vi "Stream User Timestamps to Disk.vi"(0 "fpga interface in":refnum<k20>, 5 "'stop' notifier":refnum<notifier>, 7 "base tdms file path":path, 9 "fetch size (elements)":u32=4096, 11 "error in (no error)":errorcluster) -> (4 "fpga interface out":refnum<k20>, 6 "file path out":path, 8 "gpio timestamp fifo overflow":bool, 15 "error out":errorcluster)   [LabVIEW 2023, in "GettingStarted_Common_148X_Host.lvlib"]
uses:
  GettingStarted_Common_148X_Host.lvlib
  Types/148x_Common_FPGA_Reference.ctl
  <vilib>/Utility/error.llb/Error Cluster From Error Code.vi
  <vilib>/rvi/errors/niLvFpgaAdjustHostInterfaceError.vi
  <vilib>/rvi/interface/nirviMethod/nirviMethod.xnode
  <vilib>/rvi/interface/nirviReadWriteControl/nirviReadWriteControl.xnode
  <vilib>/FPGAPlugInAG/Dynamic/niLvFpga_AcquireReadRegionFifo_Dynamic.vi
  <vilib>/rvi/errors/niLvFpgaMergeErrorWithErrorCode.vi
  NiFpgaLv.dll
  <vilib>/rvi/interface/Simulation/niFpgaSimulationCallBeginRW.vi
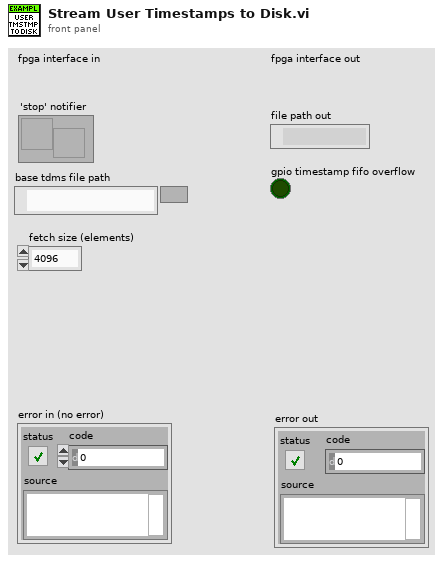
[diagram p1: front panel]
types:
  T1 = typedef "GettingStarted_Common_148X_Host.lvlib/148x_Common_FPGA_Reference.ctl" = refnum<k20>
  T2 = enum16{"open", "open or create", "create or replace", "create", "open (read-only)"}
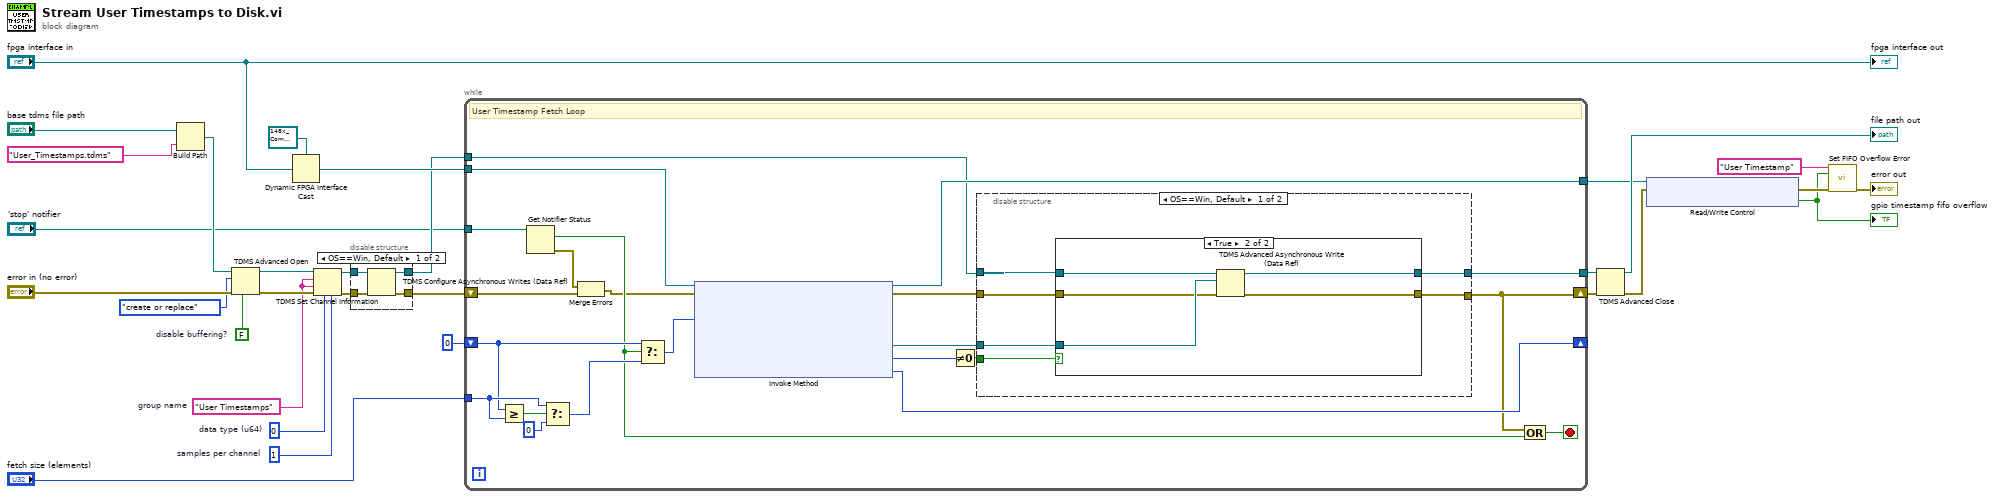
[diagram p0: block diagram]
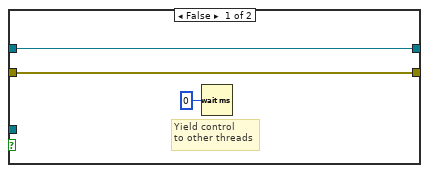
[diagram p3: hidden frame]
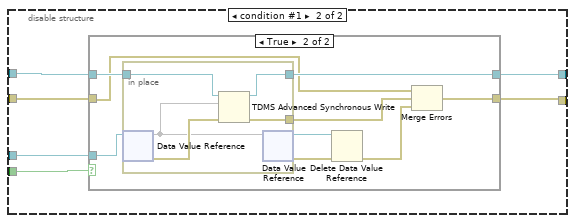
[diagram p4: hidden frame]
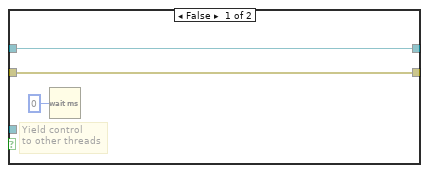
[diagram p5: hidden frame]
diagram:
  w23 = u32 1  # samples per channel
  w21 = FALSE  # disable buffering?
  w24 = u64 0  # data type (u64)
  w12 = "User Timestamps"  # group name
  n1 = Build Path(base path="base tdms file path", name or relative path="User_Timestamps.tdms") -> (appended path=w27:path)
  n2 = TDMS Advanced Open(6:w21, 8:"error in (no error)", 10:T2."create or replace" ("operation (0:open)"), 11:w27) -> (0:w15:errorcluster, 3:w16:refnum<k34>)  [unwired: 1 in, 1 out]
  n3 = Dynamic FPGA Interface Cast(Session In=T1 refnum ("FPGA VI Reference Out"), Type="fpga interface in") -> (Session Out=w19:T1)
  n4 = TDMS Set Channel Information(4:w23, 6:w24, 8:w15, 9:w12, 10:w12, 11:w16) -> (0:w9:errorcluster, 3:w10:refnum<k34>)  [unwired: 1 in]
  n5 = disable-structure shown="OS==Win, Default" {
    disable-tunnel: w9 -> [w31 w36]
    disable-tunnel: [w34 w35] -> w7
    disable-tunnel: [w33 w36] -> w8
    disable-tunnel: w10 -> [w32 w35]
    frame condition #0 (active) {
      n6 = TDMS Configure Asynchronous Writes (Data Ref)(8:w31, 11:w32) -> (0:w33:errorcluster, 3:w34:refnum<k34>)  [unwired: 2 in]
    }
    frame condition #1 {
    }
  }
  n7 = while {
    shift-right: [w47] -> w18
    shift-left: w8 -> [w38]
    tunnel: w19 -> [w42]
    shift-right: [w55] -> _
    shift-left: u32 0 ("Elements Remaining") -> [w49]
    tunnel: w7 -> [w43]
    tunnel: [w48] -> w17
    tunnel: [w56] -> w14
    tunnel: "fetch size (elements)" -> [w51]
    tunnel: "'stop' notifier" -> [w41]
    stop <- w58 stop-if-true
    # "User Timestamp Fetch Loop"
    n8 = Greater Or Equal?(x=w49, y=w51) -> (x >= y?=w54:bool)
    n9 = Get Notifier Status(notifier=w41) -> (current notification=w40:bool, error out=w37:errorcluster)  [unwired: 1 in, 3 out]
    n10 = Select(t=w51, s=w54, f=u32 0 ("Elements Remaining")) -> (s? t:f=w53:u32)
    n11 = Merge Errors(w37, w38) -> (w39:errorcluster)
    n12 = Select(t=w49, s=w40, f=w53) -> (s? t:f=w50:u32)
    n13 = xnode "Invoke Method"("FPGA VI Reference In"=w42, "error in"=w39, "Number of Elements"=w50) -> ("FPGA VI Reference Out"=w56:T1, "error out"=w44:errorcluster, "Read Region Reference"=w46:refnum<data-value>, "Elements In Region"=w57:u32, "Elements Remaining"=w55:u32)  [unwired: 1 in]
    n14 = Not Equal To 0?(x=w57) -> (x != 0?=w45:bool)
    n15 = disable-structure shown="OS==Win, Default" {
      disable-tunnel: w43 -> [w62 w78]
      disable-tunnel: w44 -> [w61 w77]
      disable-tunnel: w46 -> [w60 w76]
      disable-tunnel: w45 -> [w59 w75]
      disable-tunnel: [w64 w74] -> w48
      disable-tunnel: [w63 w73] -> w47
      frame condition #0 (active) {
        n16 = case shown="True" w59 {
          tunnel: w62 -> [w66 w72]
          tunnel: [w66 w70] -> w64
          tunnel: w61 -> [w65 w68]
          tunnel: [w65 w69] -> w63
          tunnel: w60 -> [_ w71]
          frame False {
            # "Yield control\nto other threads"
            n17 = Wait (ms)(milliseconds to wait=u32 0) -> ()  [unwired: 1 out]
          }
          frame True {
            n18 = TDMS Advanced Asynchronous Write (Data Ref)(8:w68, 10:w71, 11:w72) -> (0:w69:errorcluster, 3:w70:refnum<k34>)  [unwired: 1 in]
          }
        }
      }
      frame condition #1 {
        n19 = case shown="True" w75 {
          tunnel: w78 -> [w80 w89]
          tunnel: [w80 w86] -> w74
          tunnel: w77 -> [w79 w85]
          tunnel: [w79 w82] -> w73
          tunnel: w76 -> [_ w90]
          frame False {
            # "Yield control\nto other threads"
            n20 = Wait (ms)(milliseconds to wait=u32 0) -> ()  [unwired: 1 out]
          }
          frame True {
            n21 = in-place {
              in-place-border: w89 -> [w95]
              in-place-border: [w92] -> w84
              in-place-border: [w91] -> w86
              n22 = in-place-dvr #1(w90) -> (w93:u64[], w94:errorcluster)
              n23 = TDMS Advanced Synchronous Write(8:w94, 10:w93, 11:w95) -> (0:w92:errorcluster, 3:w91:refnum<k34>)
              n24 = in-place-dvr #1(w93) -> (w87:refnum<data-value>, w88:errorcluster)
            }
            n25 = Delete Data Value Reference(data value reference=w87, error in=w88) -> (error out=w83:errorcluster)  [unwired: 1 out]
            n26 = Merge Errors(w85, w84, w83) -> (w82:errorcluster)
          }
        }
      }
    }
    n27 = Compound Arithmetic op=OR(w47, w40) -> (w58:bool)
  }
  n28 = TDMS Advanced Close(8:w18, 11:w17) -> (0:w11:errorcluster, 3:→"file path out":path)  [unwired: 2 in]
  n29 = xnode "Read/Write Control"("FPGA VI Reference In"=w14, "error in"=w11) -> ("error out"=w6:errorcluster, "user timestamp fifo overflow"=w3:bool)  [unwired: 1 out]
  "gpio timestamp fifo overflow" <- w3
  n30 = call "Set FIFO Overflow Error.vi"("fifo name"="User Timestamp", "overflow"=w3, "error in (no error)"=w6) -> ("error out"=→"error out":errorcluster)  [unwired: 12 in]
  "fpga interface out" <- "fpga interface in"
